vi "Drive for Time.vi"(6 "Synchronization":enum16{"Start", "Wait"}(ring), 7 "Description":string, 8 "Command Info In":T1, 9 "Seconds":dbl, 10 "Right Speed":dbl, 11 "Left Speed":dbl) -> (0 "Command Info Out":T1)   [LabVIEW 2019]
doc: "This VI sets the motors to run for a given number of seconds. It optionally synchronizes with the completion of the command."
uses:
  <vilib>/Rock Robotics/WPI/Framework/Command Status Info.ctl
  <vilib>/Rock Robotics/WPI/Framework/Completion Status.ctl
  <vilib>/Rock Robotics/WPI/Framework/Completion Notifier.ctl
  Implementation/Drive Setpoints.ctl
  Implementation/Drive Operations.ctl
  Dawgma Programming Library/Controls/PurePursuit/RobotNeededPathData.ctl
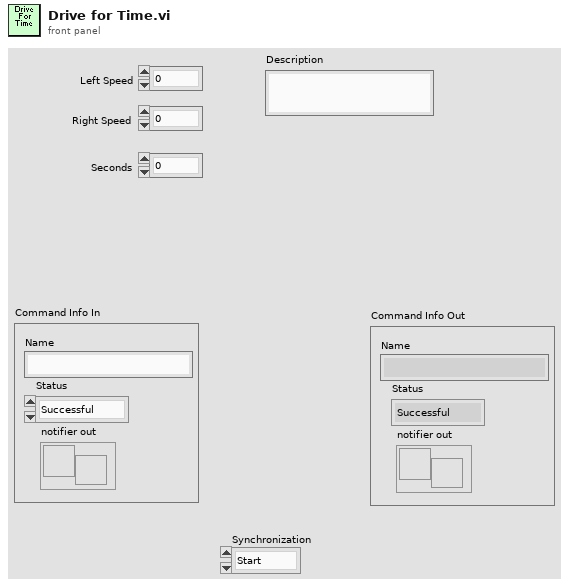
[diagram p1: front panel]
types:
  T1 = typedef "Command Status Info.ctl" = cluster{"Name":string, "Status":T2, "notifier out":T3}
  T2 = typedef "Completion Status.ctl" = enum16{"Successful", "Aborted", "Incomplete"}
  T3 = typedef "Completion Notifier.ctl" = refnum<notifier>
  T4 = typedef "Drive Setpoints.ctl" = cluster{"Operation":T5, "Left Setpoint":dbl, "Right Setpoint":dbl, "Duration":dbl, "Distance":dbl, "RobotNeededPathData":T6, "PathPath":string}
  T5 = typedef "Drive Operations.ctl" = enum16{"Reserve", "Read Current", "Immediate", "Drive for Time", "Drive for Distance", "Drive Path", "Pure Pursuit Test"}
  T6 = typedef "RobotNeededPathData.ctl" = cluster{"Path":cluster{dbl, dbl}[], "MaxVel":dbl, "MaxAccel":dbl, "Backwards?":bool, "PointSpacing":dbl, "LookaheadDist":dbl, "Speed/Curve":dbl, "SlowDistanceAtEnd":dbl, "SlowSpeed":dbl, "MaxDeAccel":dbl}
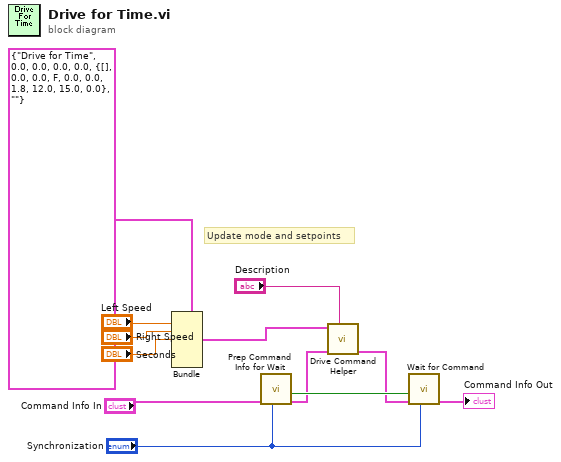
[diagram p0: block diagram]
diagram:
  # "Update mode and setpoints"
  n1 = Bundle(cluster=T4 {"Operation"=enum."Drive for Time", "Left Setpoint"=0.0, "Right Setpoint"=0.0, "Duration"=0.0, "Distance"=0.0, "RobotNeededPathData"={"Path"=[], "MaxVel"=0.0, "MaxAccel"=0.0, "Backwards?"=FALSE, "PointSpacing"=0.0, "LookaheadDist"=0.0, "Speed/Curve"=1.8, "SlowDistanceAtEnd"=12.0, "SlowSpeed"=15.0, "MaxDeAccel"=0.0}, "PathPath"=""} ("SubSystem Data"), "Left Setpoint"="Left Speed", "Right Setpoint"="Right Speed", "Duration"="Seconds") -> (w4:T4)  [unwired: 4 in]
  n2 = call <vilib>:"Prep Command Info for Wait.vi"("Synchronication"="Synchronization", "Command Info"="Command Info In") -> ("Command Info"=w8:T1, "Allocated"=w9:bool)  [unwired: 8 in]
  n3 = call "Drive Command Helper.vi"("Description"="Description", "Command Info In"=w8, "SubSystem Data"=w4) -> ("Command Info Out"=w5:T1)  [unwired: 6 in, 2 out]
  n4 = call <vilib>:"Wait for Command.vi"("Synchronication"="Synchronization", "Command Info in"=w5, "Allocated"=w9) -> ("Command Info out"=→"Command Info Out":T1)  [unwired: 8 in]
